vi "Bkgnd_place_names.vi"(1 "Numeric":i32) -> (0 "Array":string[](array[string]))   [LabVIEW 2010]
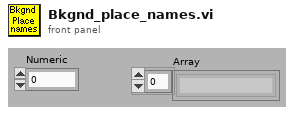
[diagram p1: front panel]
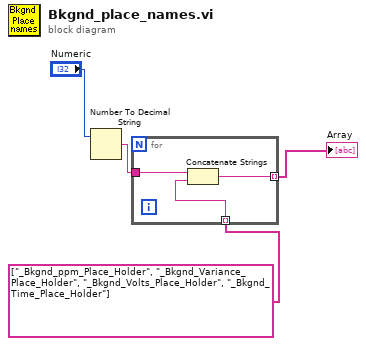
[diagram p0: block diagram]
diagram:
  n1 = Number To Decimal String(number="Numeric") -> (decimal integer string=w2:string)  [unwired: 1 out]
  n2 = for {
    tunnel: string[] ["_Bkgnd_ppm_Place_Holder", "_Bkgnd_Variance_Place_Holder", "_Bkgnd_Volts_Place_Holder", "_Bkgnd_Time_Place_Holder"] -> [w7] mode=indexing
    tunnel: w2 -> [w6]
    tunnel: [w5] -> w4 mode=indexing
    n3 = Concatenate Strings(w6, w7) -> (w5:string)
  }
  "Array" <- w4
